vi "testErrorMessageContainsCustomCaller.vi"() -> ()   [LabVIEW 2017, in "Transparent Assertions.Tests.lvlib" / "ExpectationFailedError.lvlib"]
uses:
  ExpectationFailedError.lvlib
  src/Transparent Assertions/Transparent Assertions.lvlib
panel:
  out "error out":errorcluster
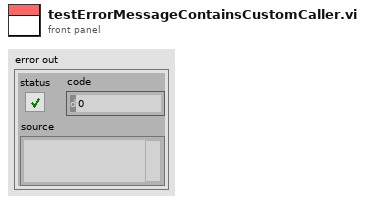
[diagram p1: front panel]
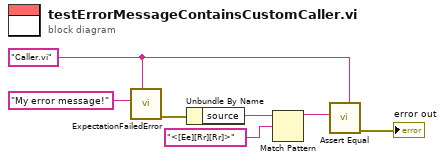
[diagram p0: block diagram]
diagram:
  w1 = "Caller.vi"
  n1 = call "ExpectationFailedError.vi"("Source (caller)"=w1, "Message"="My error message!") -> ("error out"=w5:errorcluster)  [unwired: 9 in]
  n2 = Unbundle By Name(w5) -> ("source"=w4:string)
  n3 = Match Pattern(string=w4, regular expression="<[Ee][Rr][Rr]>") -> (before substring=w2:string)  [unwired: 1 in, 3 out]
  n4 = call "Assert Equal.vi"("Expected"=w1, "Actual"=w2) -> ("error out"=→"error out":errorcluster)  [unwired: 9 in]
